vi "Send serial to caller.vi"(8 "error in (no error)":errorcluster, 10 "Serial":string, 11 "Domino Laser module Class in":refnum<class "Domino Laser module Class.lvclass">) -> (0 "error out":errorcluster, 3 "Domino Laser module Class out":refnum<class "Domino Laser module Class.lvclass">)   [LabVIEW 2015, in "Domino LM.lvlib" / "Domino Laser module Class.lvclass"]
uses:
  CTRLS/Domino Laser module Class.lvclass
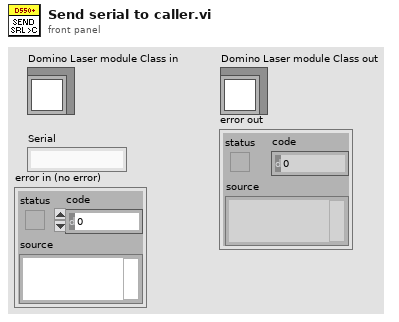
[diagram p1: front panel]
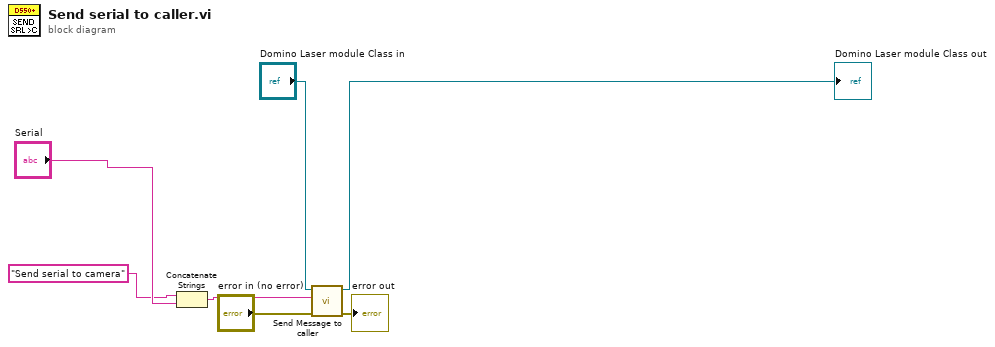
[diagram p0: block diagram]
diagram:
  n1 = Concatenate Strings("Send serial to camera" ("Message"), "Serial") -> (w3:string)
  n2 = call "Send Message to caller.vi"("error in (no error)"="error in (no error)", "Message Data"=w3, "Domino Laser module Class in"="Domino Laser module Class in") -> ("error out"=→"error out":errorcluster, "Domino Laser module Class out"=→"Domino Laser module Class out":refnum<class "Domino Laser module Class.lvclass">)  [unwired: 7 in]
